vi "Wait-for-deposition-end.vi"(8 "error in (no error)":errorcluster, 11 "Object ref in":T1) -> (0 "error out":errorcluster, 1 "Succes?":bool, 3 "Object ref out":T1)   [LabVIEW 2013, in "SLMControl.lvlib" / "SC-Main.lvclass"]
uses:
  SC-Main.lvclass
  Object-reference.ctl
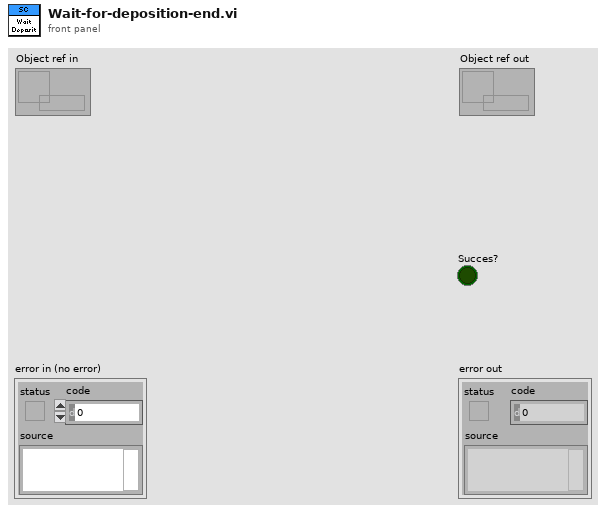
[diagram p1: front panel]
types:
  T1 = typedef "SLMControl.lvlib/SC-Main.lvclass/Object-reference.ctl" = refnum<data-value>
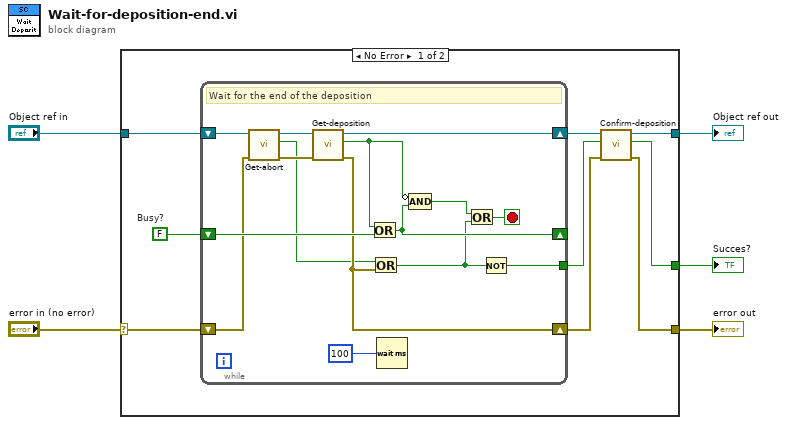
[diagram p0: block diagram]
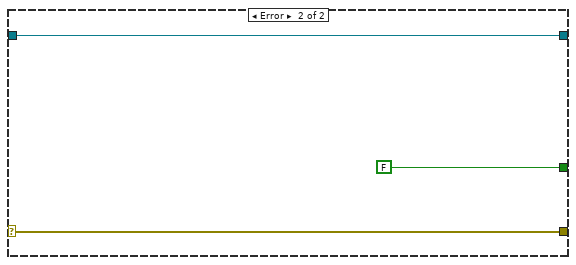
[diagram p2: hidden frame]
diagram:
  n1 = case shown="No Error" "error in (no error)" {
    selector: "error in (no error)" -> [w13 w32]
    tunnel: [w7 w32] -> w4
    tunnel: [w6 w31] -> w2
    tunnel: "Object ref in" -> [w14 w31]
    tunnel: [w9 FALSE] -> w1
    frame No Error {
      w11 = FALSE  # Busy?
      n2 = while {
        shift-right: [w21] -> w8
        shift-left: w13 -> [w25]
        shift-right: [w27] -> w12
        shift-left: w14 -> [w29]
        shift-right: [w23] -> _
        shift-left: w11 -> [w26]
        tunnel: [w16] -> w10
        stop <- w18 stop-if-true
        # "Wait for the end of the deposition"
        n3 = call "Get-abort.vi"("error in (no error)"=w25, "Object ref in"=w29) -> ("error out"=w24:errorcluster, "Abort"=w20:bool, "Object ref out"=w28:T1)  [unwired: 7 in]
        n4 = call "Get-deposition.vi"("error in (no error)"=w24, "Object ref in"=w28) -> ("error out"=w21:errorcluster, "Depositing?"=w22:bool, "Object ref out"=w27:T1)  [unwired: 7 in]
        n5 = Or(x=w22, y=w26) -> (x .or. y?=w23:bool)
        n6 = Or(x=w20, y=w21) -> (x .or. y?=w17:bool)
        n7 = Wait (ms)(milliseconds to wait=u32 100) -> ()  [unwired: 1 out]
        n8 = Compound Arithmetic op=AND(invert w22, w23) -> (w19:bool)
        n9 = Or(x=w19, y=w17) -> (x .or. y?=w18:bool)
        n10 = Not(x=w17) -> (.not. x?=w16:bool)
      }
      n11 = call "Confirm-deposition.vi"("error in (no error)"=w8, "Succes? in"=w10, "Data Value Reference in"=w12) -> ("error out"=w7:errorcluster, "Succes?"=w9:bool, "Data Value Reference out"=w6:T1)  [unwired: 6 in]
    }
    frame Error {
    }
  }
  "error out" <- w4
  "Object ref out" <- w2
  "Succes?" <- w1
